vi "Marvin.vi"() -> ()   [LabVIEW 2017]
uses:
  PCAN_Driver/ControlCAN.llb/CAN Channel.ctl
  PCAN_Driver/ControlCAN.llb/DevType.ctl
  PCAN_Driver/ControlCAN.llb/VCI_INIT_CONFIG.ctl
  PCAN_Driver/ControlCAN.llb/InitFlag.ctl
  PCAN_Driver/ControlCAN.llb/Fliter.ctl
  PCAN_Driver/ControlCAN.llb/Mode.ctl
  <vilib>/Utility/miscctls.llb/LVMinMaxIncTypeDef.ctl
  PCAN_Driver/ControlCAN.llb/VCI_CAN_OBJ.ctl
  PCAN_Driver/ControlCAN.lvlib
panel:
  in  "Numeric":i32=100
  in  "Help Button":bool
  in  "Clear Monitor":bool
  out "Array":u64[][](array[numeric]) format="%016x"
  out "Waveform Chart":dbl[](graph)
  out "Ambient Over temp":bool
  out "Ambient Sensor temp":bool
  out "Ambient Temperature":dbl
  in  "Motor Over Temp":bool
  in  "Speed control":bool
  out "Unit Adress":string
  in  "Serial Send":bool
  in  "Index":u16(ring) items=["1"=1, "2"=2, "3"=3]
  out "read buffer":string
  in  "SetGet":enum16{"Get", "Set"}(ring)
  in  "Function":T1(ring)
  in  "Value":dbl
  in  "Value 1/2":enum16{"1", "2"}(ring)
  out "Msg Count":u32
  in  "Param to Set":u16(ring) items=["EBAY 5F"=95, "AHU 3F"=63, "AHU 2F"=47]
  out "UUT":u8
  out "Horizontal Progress Bar":i32(slide) min=0 max=48 scale=0.0..50.0
  in  "Set Param.":bool
  in  "Serial Monitor":bool caption="Graph Button"
  in  "Serial Com":bool
  in  "VISA resource name":refnum<visa-resource-name>="COM6"
  out "Serial Status":bool
  in  "Graph Button":bool
  in  "Refresh Button":bool
  out "Data Send":u64 format="%016x"
  in  "Motor Speed RPM":u16
  out "Under voltage/Over voltage":bool
  out "Speed error":bool
  out "Derated drive temp":bool
  out "Motor Over temperature":bool
  out "Commutation err":bool
  out "Motor Sensor temp Fauilre":bool
  out "Drive Over temperature":bool
  out "Drive Sensor temp Failure":bool
  out "Motor Phase Current RMS":dbl
  out "ECS State":u16
  out "Motor Speed RPM":dbl
  out "Motor Stator Temp.":dbl
  out "Power transistor Heat sink Temp.":dbl
  out "DC Current":dbl
  out "DC Voltage":dbl
  in  "Can Send":bool
  in  "Stop":bool
  out "Config_CANAT":T8 {"DevType" items=["USB-CAN"=3, "USB-CAN2"=4]; "CanIndex" items=["通道1", "通道2"]; "VCI_INIT_CONFIG"."Fliter" items=["接收所有类型"=3, "只接收标准帧"=4, "只接收扩展帧"=7]; "VCI_INIT_CONFIG"."Mode" items=["正常工作", "自测模式（环回）", "仅侦听模式"]; "VCI_INIT_CONFIG"."InitFlag" items=["使用Flash参数", "使用界面设置参数"]}
  in  "Channel 2":T3 caption="Channel" items=["Channel 1", "Channel 2"]
  out "CAN Status":bool
  # "ver 1.5"
  # "Marvin"
  # "REDLER TECHNOLOGIES LTD"
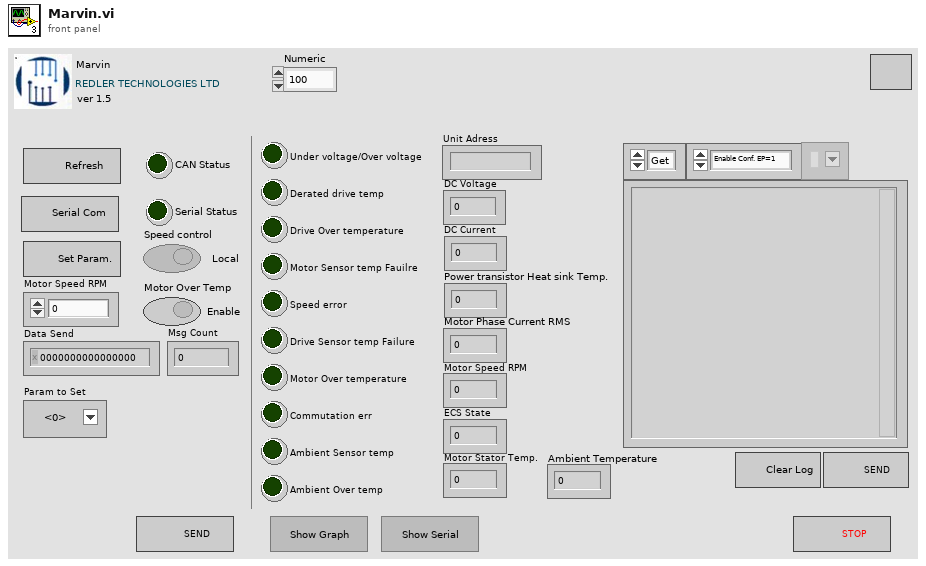
[diagram p1: front panel]
types:
  T1 = enum16{"Enable Conf. EP=1", "Serial Number", "Temperature", "Unit Adress", "Calibration", "Velocity", "Version"}
  T2 = typedef "ControlCAN.lvlib/DevType.ctl" = u32
  T3 = typedef "ControlCAN.lvlib/CAN Channel.ctl" = u32
  T4 = typedef "ControlCAN.lvlib/VCI_INIT_CONFIG.ctl" = cluster{"AccCode":u32, "AccMask":u32, "InitFlag":T5, "Fliter":T6, "Timing0":u8, "Timing1":u8, "Mode":T7}
  T5 = typedef "ControlCAN.lvlib/InitFlag.ctl" = u32
  T6 = typedef "ControlCAN.lvlib/Fliter.ctl" = u8
  T7 = typedef "ControlCAN.lvlib/Mode.ctl" = u8
  T8 = cluster{"DevType":T2, "DevIndex":u32, "CanIndex":T3, "VCI_INIT_CONFIG":T4}
  T9 = cluster{"ID":u32, "MSGTYPE":u8, "LEN":u8, "aDATA":u8[]}[]
  T10 = cluster{"ID":u32, "MSGTYPE":u8, "LEN":u8, "aDATA":u8[]}
  T11 = enum8{"Enabled", "Disabled", "Disabled and Grayed Out"}
  T12 = typedef "LVMinMaxIncTypeDef.ctl" = cluster{"Minimum":dbl, "Maximum":dbl, "Increment":dbl}
  T13 = enum32{"Invalid", "Standard", "Closed", "Hidden", "Minimized", "Maximized"}
  T14 = typedef "ControlCAN.lvlib/VCI_CAN_OBJ.ctl" = cluster{"ID":u32, "TimeStamp":u32, "TimeFlag":u8, "SendType":u8, "RemoteFlag":u8, "ExternFlag":u8, "DataLen":u8, "Data":u8[], "Reserved":u8[]}
  T15 = cluster{"Type":enum16{"接收", "发送"}, "Channel":T3, "Time":timestamp, "VCI_CAN_OBJ":T14}[]
  T16 = cluster{"Type":enum16{"接收", "发送"}, "Channel":T3, "Time":timestamp, "VCI_CAN_OBJ":T14}
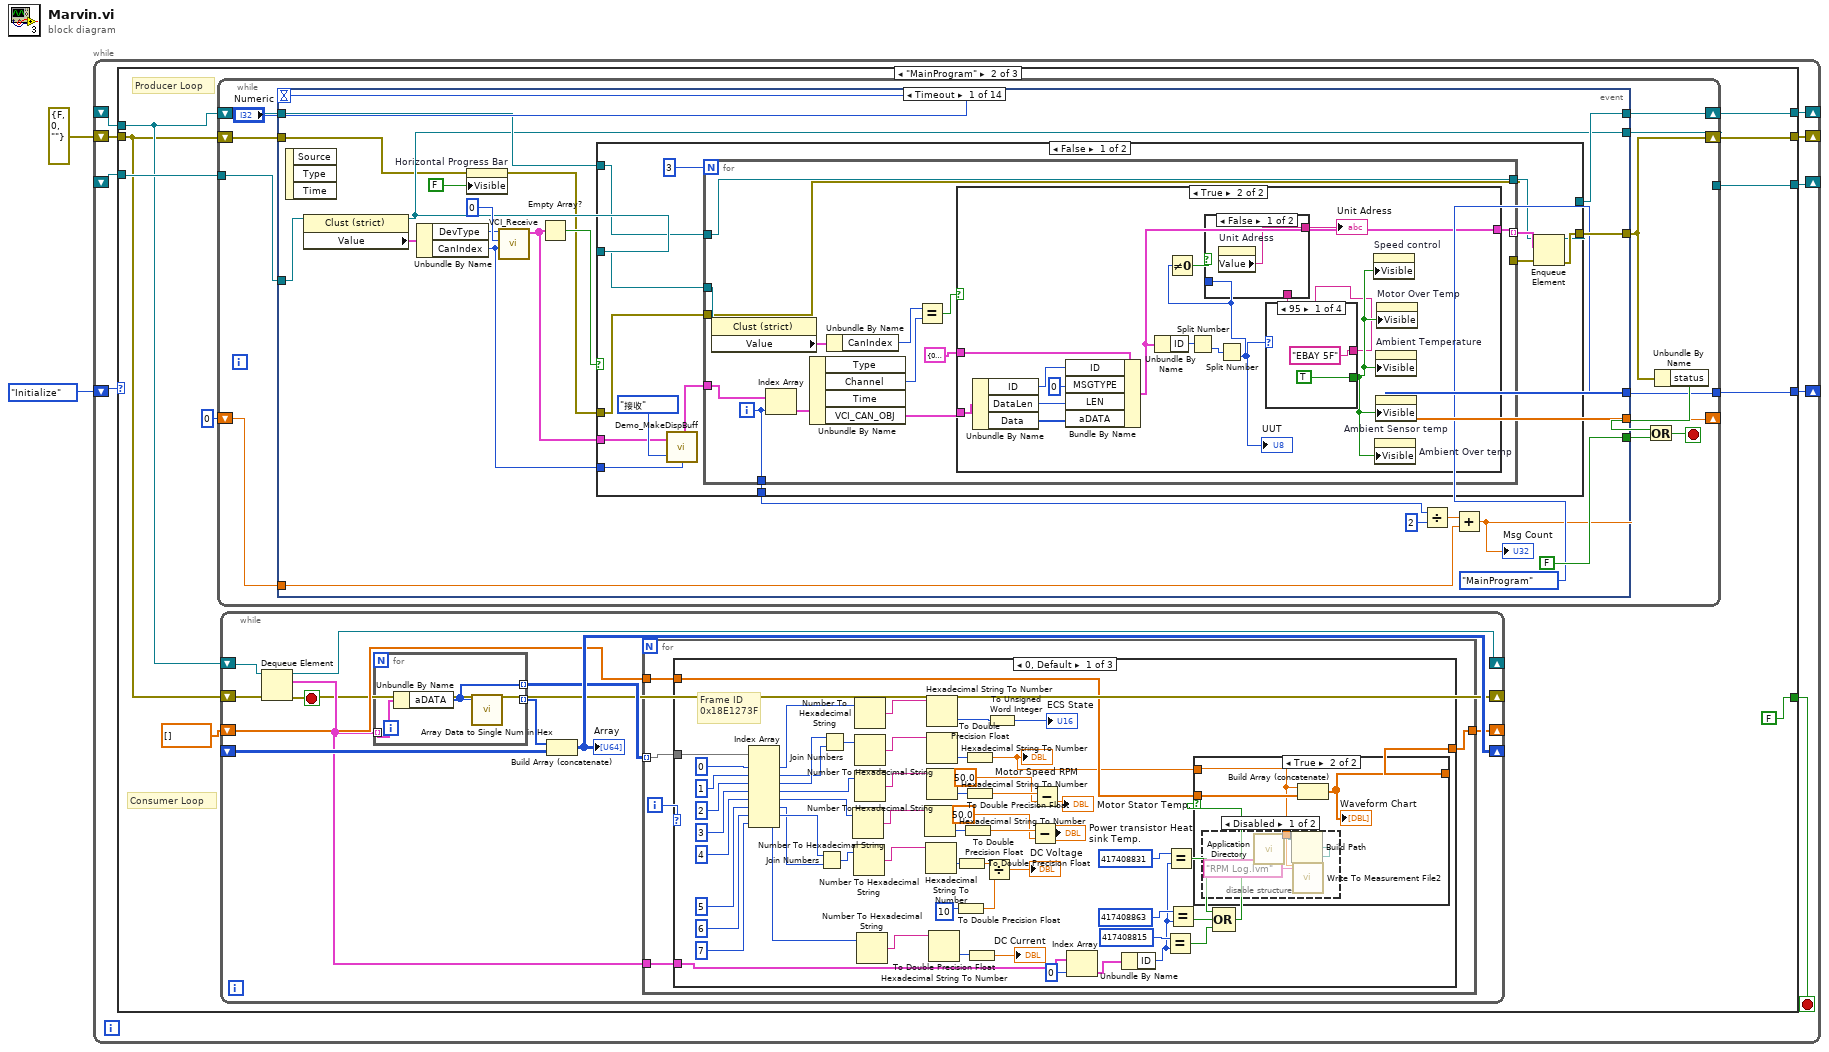
[diagram p0: block diagram]
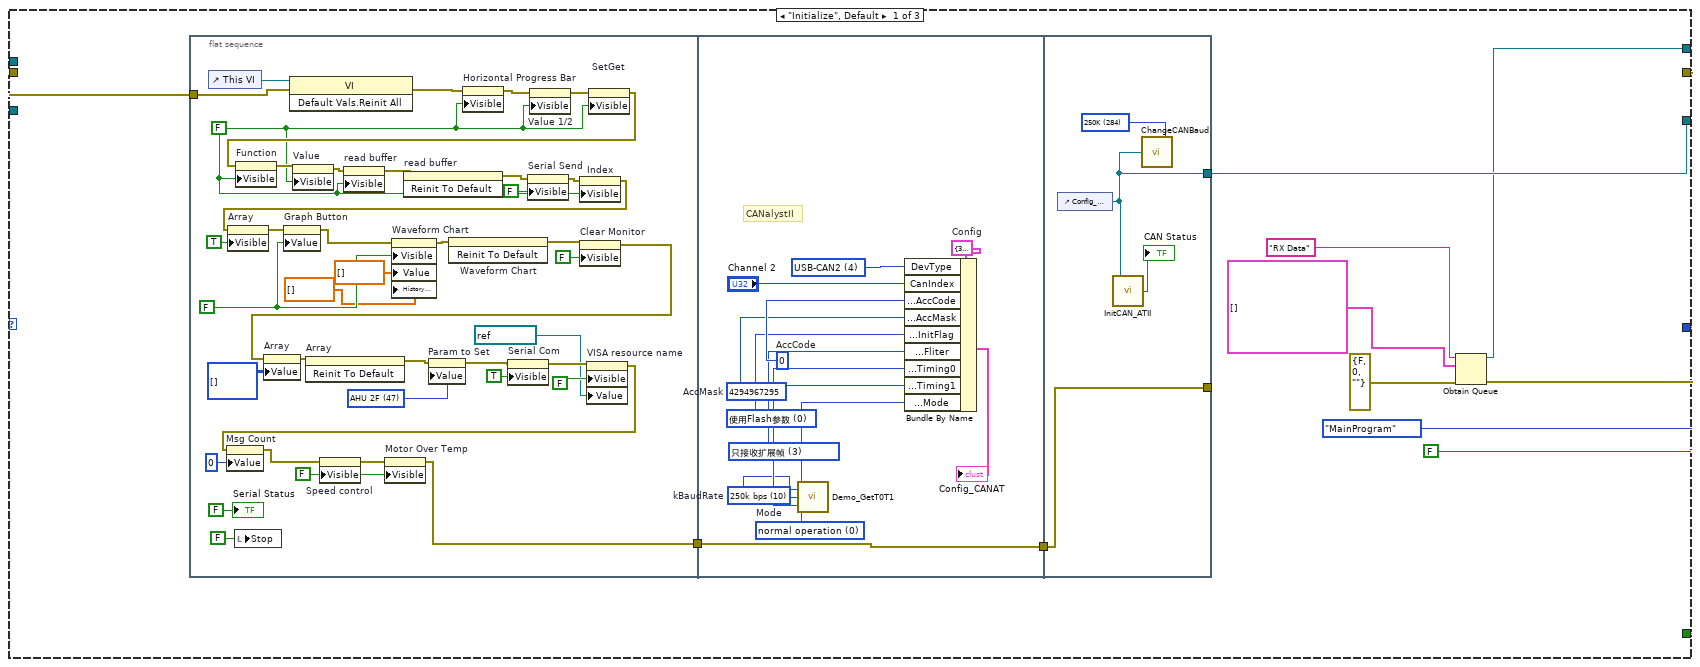
[diagram p2: hidden frame]
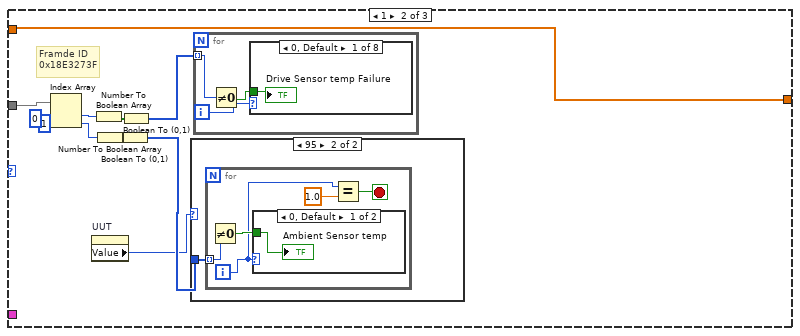
[diagram p5: hidden frame]
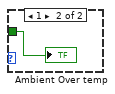
[diagram p7: hidden frame]
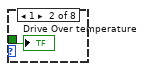
[diagram p8: hidden frame]
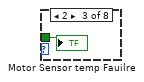
[diagram p9: hidden frame]
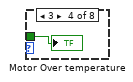
[diagram p10: hidden frame]
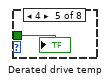
[diagram p11: hidden frame]
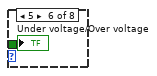
[diagram p12: hidden frame]
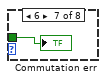
[diagram p13: hidden frame]
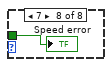
[diagram p14: hidden frame]
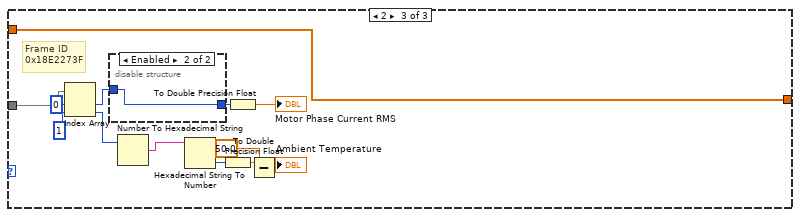
[diagram p15: hidden frame]
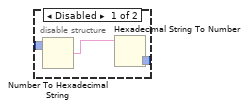
[diagram p16: hidden frame]
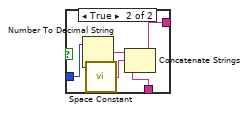
[diagram p18: hidden frame]
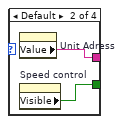
[diagram p19: hidden frame]
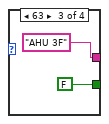
[diagram p20: hidden frame]
diagram:
  n1 = while {
    shift-right: [w6] -> _
    shift-left: enum16{"Stop", "MainProgram", "Initialize"}."Initialize" -> [w11]
    shift-right: [w10] -> _
    shift-left: _ -> [w9]
    shift-right: [w8] -> _
    shift-left: _ -> [w5]
    shift-right: [w7] -> _
    shift-left: errorcluster {"status"=FALSE, "code"=0, "source"=""} ("error out") -> [w4]
    stop <- w3 stop-if-true
    n2 = case shown="\"MainProgram\"" w11 {
      tunnel: [w22 w87 w917] -> w10
      tunnel: w9 -> [_ w90 w917]
      tunnel: [w18 w89 w918] -> w8
      tunnel: [w17 w88 w919] -> w7
      tunnel: [enum16{"Stop", "MainProgram", "Initialize"}."MainProgram" w86 enum16{"Stop", "MainProgram", "Initialize"}."Stop"] -> w6
      tunnel: w5 -> [_ w85 w918]
      tunnel: w4 -> [w15 w84 w920]
      tunnel: [FALSE ("Stop") FALSE ("Stop") w916] -> w3
      frame "Initialize", Default {
        n3 = flat-sequence {
          tunnel: w15 -> [w36]
          tunnel: [w32] -> w13
          tunnel: [w64] -> w14
          tunnel: w13 -> [w64]
          tunnel: [w78] -> w22
          tunnel: w14 -> [w77]
          tunnel: [w77] -> _
          frame #0 {
            w31 = FALSE ("Visible")
            w49 = u16 47 items=["EBAY 5F"=95, "AHU 3F"=63, "AHU 2F"=47] ("Param to Set")
            w26 = FALSE ("Visible")
            w55 = FALSE ("Graph Button")
            n4 = control-ref of="This VI"() -> (w63:refnum<vi>)
            n5 = local write "Stop"(FALSE ("Stop")) -> ()
            n6 = invoke class="VI" method="Default Vals.Reinit All"(reference=w63, error in=w36) -> (error out=w35:errorcluster)  [unwired: 1 in, 2 out]
            n7 = property on="Horizontal Progress Bar" class="Slide (strict)"(error in=w35, "Visible"=w26) -> (error out=w47:errorcluster)  [unwired: 1 in, 1 out]
            n8 = property on="Value 1/2" class="Enum (strict)"(error in=w47, "Visible"=w26) -> (error out=w46:errorcluster)  [unwired: 1 in, 1 out]
            n9 = property on="SetGet" class="Enum (strict)"(error in=w46, "Visible"=w26) -> (error out=w45:errorcluster)  [unwired: 1 in, 1 out]
            n10 = property on="Function" class="Enum (strict)"(error in=w45, "Visible"=w26) -> (error out=w44:errorcluster)  [unwired: 1 in, 1 out]
            n11 = property on="Value" class="DigNum (strict)"(error in=w44, "Visible"=w26) -> (error out=w43:errorcluster)  [unwired: 1 in, 1 out]
            n12 = property on="read buffer" class="Str"(error in=w43, "Visible"=w26) -> (error out=w28:errorcluster)  [unwired: 1 in, 1 out]
            n13 = invoke on="read buffer" class="Str" method="Reinit To Default"(error in=w28) -> (error out=w27:errorcluster)  [unwired: 2 in, 2 out]
            n14 = property on="Serial Send" class="Bool"(error in=w27, "Visible"=FALSE) -> (error out=w42:errorcluster)  [unwired: 1 in, 1 out]
            n15 = property on="Index" class="Ring (strict)"(error in=w42, "Visible"=w26) -> (error out=w41:errorcluster)  [unwired: 1 in, 1 out]
            n16 = property on="Array" class="Arr (strict)"(error in=w41, "Visible"=TRUE) -> (error out=w40:errorcluster)  [unwired: 1 in, 1 out]
            n17 = property on="Graph Button" class="Bool (strict)"(error in=w40, "Value"=w55) -> (error out=w39:errorcluster)  [unwired: 1 in, 1 out]
            n18 = property on="Waveform Chart" class="WFChart (strict)"(error in=w39, "Visible"=w55, "Value"=dbl[] [] ("Waveform Chart"), "History Data"=dbl[] []) -> (error out=w58:errorcluster)  [unwired: 1 in, 1 out]
            n19 = invoke on="Waveform Chart" class="WFChart (strict)" method="Reinit To Default"(error in=w58) -> (error out=w25:errorcluster)  [unwired: 2 in, 2 out]
            n20 = property on="Clear Monitor" class="Bool"(error in=w25, "Visible"=FALSE) -> (error out=w24:errorcluster)  [unwired: 1 in, 1 out]
            n21 = property on="Array" class="Arr (strict)"(error in=w24, "Value"=u64[][] [] ("Array")) -> (error out=w30:errorcluster)  [unwired: 1 in, 1 out]
            n22 = invoke on="Array" class="Arr (strict)" method="Reinit To Default"(error in=w30) -> (error out=w29:errorcluster)  [unwired: 2 in, 2 out]
            n23 = property on="Param to Set" class="Ring (strict)"(error in=w29, "Value"=w49) -> (error out=w38:errorcluster)  [unwired: 1 in, 1 out]
            n24 = property on="Serial Com" class="Bool"(error in=w38, "Visible"=TRUE) -> (error out=w60:errorcluster)  [unwired: 1 in, 1 out]
            n25 = property on="VISA resource name" class="VISAName"(error in=w60, "Visible"=FALSE, "Value"=refnum<visa-resource-name> "COM1" ("VISA resource name")) -> (error out=w37:errorcluster)  [unwired: 1 in, 1 out]
            n26 = property on="Msg Count" class="DigNum (strict)"(error in=w37, "Value"=u32 0 ("Msg Count")) -> (error out=w34:errorcluster)  [unwired: 1 in, 1 out]
            n27 = property on="Speed control" class="Bool (strict)"(error in=w34, "Visible"=w31) -> (error out=w33:errorcluster)  [unwired: 1 in, 1 out]
            n28 = property on="Motor Over Temp" class="Bool (strict)"(error in=w33, "Visible"=w31) -> (error out=w32:errorcluster)  [unwired: 1 in, 1 out]
            "Serial Status" <- FALSE ("Serial Status")
          }
          frame #1 {
            w68 = u32 4294967295  # AccMask
            w67 = T5 0 items=["使用Flash参数", "使用界面设置参数"] ("InitFlag")
            w65 = T7 0 items=["normal operation", "Listen-only mode", "test mode"]  # Mode
            w66 = T6 3 items=["接收所有类型"=1, "只接收标准帧"=2, "只接收扩展帧"=3] ("Fliter")
            w72 = u8 10 items=["5k bps"=1, "10k bps"=2, "20k bps"=3, "40k bps"=4, "50k bps"=5, "80k bps"=6, "100k bps"=7, "125k bps"=8, "200k bps"=9, "250k bps"=10, "400k bps"=11, "500k bps"=12, "666k bps"=13, "800k bps"=14, "1000k bps"=15, "33.33k bps"=16, "66.66k bps"=17, "83.33k bps"=18]  # kBaudRate
            w69 = u32 0  # AccCode
            w70 = T2 4 items=["USB-CAN"=3, "USB-CAN2"=4] ("DevType")
            w71 = T8 {"DevType"=3, "DevIndex"=0, "CanIndex"=0, "VCI_INIT_CONFIG"={"AccCode"=0, "AccMask"=0, "InitFlag"=1, "Fliter"=7, "Timing0"=0, "Timing1"=0, "Mode"=0}}  # Config
            # "CANalystII"
            n29 = call "Demo_GetT0T1.vi"("kBaudRate"=w72) -> ("Timing0"=w74:u8, "Timing1"=w75:u8)
            n30 = Bundle By Name(cluster=w71, "DevType"=w70, "CanIndex"="Channel 2", "VCI_INIT_CONFIG.AccCode"=w69, "VCI_INIT_CONFIG.AccMask"=w68, "VCI_INIT_CONFIG.InitFlag"=w67, "VCI_INIT_CONFIG.Fliter"=w66, "VCI_INIT_CONFIG.Timing0"=w74, "VCI_INIT_CONFIG.Timing1"=w75, "VCI_INIT_CONFIG.Mode"=w65) -> (→"Config_CANAT":T8)
          }
          frame #2 {
            w79 = u16 284 items=["1M"=20, "500K"=28, "250K"=284, "125K"=796, "100K"=17199, "50K"=18223, "20K"=21295, "10K"=26415, "5K"=32639] ("baud in")
            n31 = control-ref of="Config_CANAT"() -> (w78:refnum<vi>)
            n32 = call "InitCAN_ATII.vi"("Config"=w78) -> ("Sts"=→"CAN Status":bool)
            n33 = call "ChangeCANBaud.vi"("baud in"=w79, "reference"=w78) -> ()
          }
        }
        n34 = Obtain Queue(name (unnamed)="RX Data", element data type=T9 [], error in (no error)=errorcluster {"status"=FALSE, "code"=0, "source"=""}) -> (queue out=w18:refnum<queue>, error out=w17:errorcluster)  [unwired: 2 in, 1 out]
      }
      frame "MainProgram" {
        # "Consumer Loop"
        # "Producer Loop"
        n35 = while {
          shift-right: [w228] -> w88
          shift-left: w84 -> [w230]
          shift-right: [w229] -> w89
          shift-left: w85 -> [w231]
          tunnel: w90 -> [w232]
          tunnel: [w225] -> w87
          tunnel: [w224] -> w86
          shift-right: [w222] -> _
          shift-left: 0 -> [w223]
          stop <- w233 stop-if-true
          n36 = event shown="[0] Timeout" {
            selector: _ -> [_ _ _ _ _ _ _ _ _ _ _ _ _ _]
            dyn-events: _ -> [_ _ _ _ _ _ _ _ _ _ _ _ _ _]
            timeout: "Numeric" -> [_ _ _ _ _ _ _ _ _ _ _ _ _ _]
            tunnel: w232 -> [w252 w322 w332 w392 w582 w615 w662 w759 w779 w855 w875 w892 w907 w913]
            tunnel: w231 -> [w249 w323 w335 w393 w583 w616 w661 w760 w800 w856 w874 w893 w904 w910]
            tunnel: w230 -> [w241 w321 w330 w387 w585 w618 w654 w752 w799 w848 w870 w885 w903 w911]
            tunnel: [w247 w323 w335 w393 w583 w616 w661 w760 w800 w856 w874 w893 w902 w910] -> w229
            tunnel: [w246 w315 w331 w384 w581 w617 w650 w749 w799 w836 w867 w883 w900 w909] -> w228
            tunnel: [FALSE ("Stop") FALSE ("Stop") FALSE ("Stop") FALSE ("Stop") FALSE ("Stop") FALSE ("Stop") FALSE ("Stop") FALSE ("Stop") FALSE ("Stop") FALSE ("Stop") FALSE ("Stop") FALSE ("Stop") TRUE ("Stop") TRUE ("Stop")] -> w226
            tunnel: [w245 w322 w332 w392 w582 w615 w662 w759 w779 w855 w875 w892 w907 w913] -> w225
            tunnel: [enum16{"Stop", "MainProgram", "Initialize"}."MainProgram" enum16{"Stop", "MainProgram", "Initialize"}."MainProgram" enum16{"Stop", "MainProgram", "Initialize"}."MainProgram" enum16{"Stop", "MainProgram", "Initialize"}."MainProgram" enum16{"Stop", "MainProgram", "Initialize"}."MainProgram" enum16{"Stop", "MainProgram", "Initialize"}."MainProgram" enum16{"Stop", "MainProgram", "Initialize"}."MainProgram" enum16{"Stop", "MainProgram", "Initialize"}."MainProgram" enum16{"Stop", "MainProgram", "Initialize"}."MainProgram" enum16{"Stop", "MainProgram", "Initialize"}."MainProgram" enum16{"Stop", "MainProgram", "Initialize"}."MainProgram" enum16{"Stop", "MainProgram", "Initialize"}."MainProgram" enum16{"Stop", "MainProgram", "Initialize"}."Stop" enum16{"Stop", "MainProgram", "Initialize"}."Initialize"] -> w224
            tunnel: w223 -> [w240 w326 w328 w380 w579 w614 w652 w763 w765 w846 w866 w881 w899 w908]
            tunnel: [w239 w326 w328 w380 w579 w614 w652 w763 w765 w846 w866 w881 w899 w908] -> w222
            event Timeout {
              n37 = event-data() -> ()  [unwired: 1 in, 3 out]
              n38 = property class="Clust (strict)"(reference=w252) -> (reference out=w245:refnum<vi>, "Value"=w253:T8)  [unwired: 1 in, 1 out]
              n39 = Unbundle By Name(w253) -> ("DevType"=w254:T2, "CanIndex"=w250:T3)
              n40 = property on="Horizontal Progress Bar" class="Slide (strict)"(error in=w241, "Visible"=FALSE) -> (error out=w235:errorcluster)  [unwired: 1 in, 1 out]
              n41 = call "VCI_Receive.vi"("CANIndex"=w250, "DevIndex"=u32 0, "DevType"=w254) -> ("Recieve"=w248:T14[])  [unwired: 3 in, 5 out]
              n42 = Empty Array?(array=w248) -> (empty?=w251:bool)
              n43 = case shown="False" w251 {
                tunnel: w250 -> [w267 _]
                tunnel: w245 -> [w265 _]
                tunnel: w249 -> [w264 w314]
                tunnel: w235 -> [w263 w313]
                tunnel: w248 -> [w268 _]
                tunnel: [w258 w313] -> w246
                tunnel: [w257 w314] -> w247
                tunnel: [w256 0] -> w236
                frame False {
                  n44 = call "Demo_MakeDispBuff.vi"("Channel"=w267, "Type"=enum16{"接收", "发送"}."接收", "OBJs"=w268) -> ("Buffer"=w266:T15)
                  n45 = for {
                    N: 3 -> [_]
                    tunnel: w266 -> [w282]
                    tunnel: w265 -> [w281]
                    tunnel: w264 -> [w272]
                    tunnel: w263 -> [w271]
                    tunnel: [w274] -> w261 mode=indexing
                    tunnel: [w272] -> w260
                    tunnel: [w271] -> w259
                    tunnel: [w270] -> w256
                    i -> [w270]
                    n46 = property class="Clust (strict)"(reference=w281) -> ("Value"=w279:T8)  [unwired: 1 in, 2 out]
                    n47 = Index Array(array=w282, index=w270) -> (element=w275:T16)
                    n48 = Unbundle By Name(w275) -> ("Channel"=w277:T3, "VCI_CAN_OBJ"=w280:T14)  [unwired: 2 out]
                    n49 = Unbundle By Name(w279) -> ("CanIndex"=w278:T3)
                    n50 = Equal?(x=w278, y=w277) -> (x = y?=w276:bool)
                    n51 = case shown="True" w276 {
                      tunnel: w280 -> [_ w297]
                      tunnel: [w283 w293] -> w274
                      tunnel: T10 {"ID"=0, "MSGTYPE"=0, "LEN"=0, "aDATA"=[]} ("Msg") -> [w283 w292]
                      frame False {
                      }
                      frame True {
                        n52 = Unbundle By Name(w297) -> ("ID"=w291:u32, "DataLen"=w296:u8, "Data"=w294:u8[])
                        n53 = Bundle By Name(cluster=w292, "ID"=w291, "MSGTYPE"=u8 0, "LEN"=w296, "aDATA"=w294) -> (w293:T10)
                        n54 = Unbundle By Name(w293) -> ("ID"=w289:u32)
                        n55 = Split Number(x=w289) -> (lo(x)=w290:u16)  [unwired: 1 out]
                        n56 = Split Number(x=w290) -> (lo(x)=w286:u8)  [unwired: 1 out]
                        "UUT" <- w286
                        n57 = Not Equal To 0?(x=w286) -> (x != 0?=w287:bool)
                        n58 = case shown="95" w286 {
                          tunnel: ["EBAY 5F" w306 "AHU 3F" "AHU 2F"] -> w285
                          tunnel: [TRUE w307 FALSE FALSE] -> w288
                          frame 95 {
                          }
                          frame Default {
                            n59 = property on="Unit Adress" class="Str"() -> ("Value"=w306:string)  [unwired: 2 in, 2 out]
                            n60 = property on="Speed control" class="Bool (strict)"() -> ("Visible"=w307:bool)  [unwired: 2 in, 2 out]
                          }
                          frame 63 {
                          }
                          frame 47 {
                          }
                        }
                        n61 = case shown="False" w287 {
                          tunnel: w286 -> [_ w303]
                          tunnel: w285 -> [_ w300]
                          tunnel: [w298 w299] -> w284
                          frame False {
                            n62 = property on="Unit Adress" class="Str"() -> ("Value"=w298:string)  [unwired: 2 in, 2 out]
                          }
                          frame True {
                            n63 = Number To Decimal String(number=w303) -> (decimal integer string=w302:string)  [unwired: 1 in]
                            n64 = call <vilib>:"Space Constant.vi"() -> ("String"=w301:string)
                            n65 = Concatenate Strings(w302, w301, w300) -> (w299:string)
                          }
                        }
                        "Unit Adress" <- w284
                        n66 = property on="Speed control" class="Bool (strict)"("Visible"=w288) -> ()  [unwired: 2 in, 2 out]
                        n67 = property on="Ambient Over temp" class="Bool (strict)"("Visible"=w288) -> ()  [unwired: 2 in, 2 out]
                        n68 = property on="Ambient Temperature" class="DigNum (strict)"("Visible"=w288) -> ()  [unwired: 2 in, 2 out]
                        n69 = property on="Ambient Sensor temp" class="Bool (strict)"("Visible"=w288) -> ()  [unwired: 2 in, 2 out]
                        n70 = property on="Motor Over Temp" class="Bool (strict)"("Visible"=w288) -> ()  [unwired: 2 in, 2 out]
                      }
                    }
                  }
                  n71 = Enqueue Element(queue=w260, element=w261, error in (no error)=w259) -> (queue out=w257:refnum<queue>, error out=w258:errorcluster)  [unwired: 2 out]
                }
                frame True {
                }
              }
              n72 = Divide(x=w236, y=u32 2) -> (x/y=w237:dbl)
              n73 = Add(x=w237, y=w240) -> (x+y=w239:dbl)
              "Msg Count" <- w239
            }
            event "Clear Monitor": Value Change {
              n74 = event-data() -> ()  [unwired: 1 in, 6 out]
              n75 = property on="VISA resource name" class="VISAName"(error in=w321) -> (error out=w320:errorcluster, "Value"=w318:refnum<visa-resource-name>)  [unwired: 1 in, 1 out]
              n76 = call "Serial.vi"("error in (no error)"=w320, "Clear Log"=TRUE, "VISA resource name"=w318) -> ("error out"=w316:errorcluster, "read buffer"=w317:string)  [unwired: 6 in, 1 out]
              n77 = property on="read buffer" class="Str"(error in=w316, "Value"=w317) -> (error out=w315:errorcluster)  [unwired: 1 in, 1 out]
            }
            event "Serial Monitor": Value Change {
              n78 = event-data() -> ()  [unwired: 1 in, 6 out]
              n79 = property on="Serial Status" class="Bool (strict)"(error in=w330) -> (error out=w329:errorcluster, "Value"=w327:bool)  [unwired: 1 in, 1 out]
              n80 = case shown="True" w327 {
                tunnel: w329 -> [w339 w352]
                tunnel: [w337 w357] -> w331
                frame False {
                  n81 = call "Display Message to User3"("error in (no error)"=w339) -> ("error out"=w338:errorcluster)  [unwired: 9 in, 1 out]
                  n82 = property on="Serial Monitor" class="Bool (strict)"(error in=w338, "Value"=FALSE ("Serial Monitor")) -> (error out=w337:errorcluster)  [unwired: 1 in, 1 out]
                }
                frame True {
                  w344 = FALSE ("Visible")
                  w354 = FALSE ("Visible")
                  w355 = u16 1 items=["1"=1, "2"=2, "3"=3] ("Index")
                  n83 = property on="Index" class="Ring (strict)"(error in=w352, "Value"=w355) -> (error out=w351:errorcluster)  [unwired: 1 in, 1 out]
                  n84 = property on="Value 1/2" class="Enum (strict)"(error in=w351, "Visible"=w354) -> (error out=w350:errorcluster)  [unwired: 1 in, 1 out]
                  n85 = property on="Value" class="DigNum (strict)"(error in=w350, "Visible"=w354) -> (error out=w349:errorcluster)  [unwired: 1 in, 1 out]
                  n86 = property on="SetGet" class="Enum (strict)"(error in=w349, "Value"=enum16{"Get", "Set"}."Get" ("SetGet")) -> (error out=w348:errorcluster)  [unwired: 1 in, 1 out]
                  n87 = property on="Serial Send" class="Bool"(error in=w348, "Visible"=w344) -> (error out=w343:errorcluster)  [unwired: 1 in, 1 out]
                  n88 = property on="Clear Monitor" class="Bool"(error in=w343, "Visible"=w344) -> (error out=w342:errorcluster)  [unwired: 1 in, 1 out]
                  n89 = property on="Function" class="Enum (strict)"(error in=w342, "Value"=T1."Serial Number" ("Function")) -> (error out=w347:errorcluster)  [unwired: 1 in, 1 out]
                  n90 = property on="Index" class="Ring (strict)"(error in=w347, "DisabledEnum"=T11."Disabled and Grayed Out" ("Disabled")) -> (error out=w345:errorcluster)  [unwired: 1 in, 1 out]
                  n91 = case shown="True" "Serial Monitor" {
                    selector: "Serial Monitor" -> [w361 w376]
                    tunnel: w345 -> [w360 w379]
                    tunnel: [w363 w373] -> w357
                    tunnel: [FALSE TRUE] -> w341
                    frame False {
                      n92 = property on="Graph Button" class="Bool (strict)"(error in=w360) -> (error out=w359:errorcluster, "Value"=w358:bool)  [unwired: 1 in, 1 out]
                      n93 = case shown="True" w358 {
                        tunnel: [w368 w371] -> w364
                        tunnel: w359 -> [w367 w370]
                        tunnel: w361 -> [w365 _]
                        frame False {
                          n94 = Not(x=w365) -> (.not. x?=w366:bool)
                          n95 = property on="Array" class="Arr (strict)"(error in=w367, "Visible"=w366) -> (error out=w368:errorcluster)  [unwired: 1 in, 1 out]
                        }
                        frame True {
                          n96 = property on="Array" class="Arr (strict)"(error in=w370, "Visible"=FALSE) -> (error out=w371:errorcluster)  [unwired: 1 in, 1 out]
                        }
                      }
                      n97 = property on="Serial Monitor" class="Bool (strict)"(error in=w364, "Value"=w361) -> (error out=w363:errorcluster)  [unwired: 1 in, 1 out]
                    }
                    frame True {
                      n98 = Not(x=w376) -> (.not. x?=w372:bool)
                      n99 = property on="Array" class="Arr (strict)"(error in=w379, "Visible"=w372) -> (error out=w378:errorcluster)  [unwired: 1 in, 1 out]
                      n100 = property on="Serial Monitor" class="Bool (strict)"(error in=w378, "Value"=w376) -> (error out=w375:errorcluster)  [unwired: 1 in, 1 out]
                      n101 = property on="Graph Button" class="Bool (strict)"(error in=w375, "Value"=w372) -> (error out=w374:errorcluster)  [unwired: 1 in, 1 out]
                      n102 = property on="Waveform Chart" class="WFChart (strict)"(error in=w374, "Visible"=w372) -> (error out=w373:errorcluster)  [unwired: 1 in, 1 out]
                    }
                  }
                  n103 = property on="SetGet" class="Enum (strict)"("Visible"=w341) -> ()  [unwired: 2 in, 2 out]
                  n104 = property on="Index" class="Ring (strict)"("Visible"=w341) -> ()  [unwired: 2 in, 2 out]
                  n105 = property on="Function" class="Enum (strict)"("Visible"=w341) -> ()  [unwired: 2 in, 2 out]
                  n106 = property on="Clear Monitor" class="Bool"("Visible"=w341) -> ()  [unwired: 2 in, 2 out]
                  n107 = property on="Serial Send" class="Bool"("Visible"=w341) -> ()  [unwired: 2 in, 2 out]
                  n108 = property on="read buffer" class="Str"("Visible"=w341) -> ()  [unwired: 2 in, 2 out]
                }
              }
            }
            event "Serial Send": Value Change {
              n109 = event-data() -> ()  [unwired: 1 in, 6 out]
              n110 = property on="read buffer" class="Str"(error in=w387) -> (error out=w386:errorcluster, "Text.Scroll Position"=w383:u32)  [unwired: 1 in, 1 out]
              n111 = property on="VISA resource name" class="VISAName"() -> ("Value"=w394:refnum<visa-resource-name>)  [unwired: 2 in, 2 out]
              n112 = case shown="\"Get\", Default" "SetGet" {
                tunnel: "Function" -> [w401 w486]
                tunnel: w394 -> [w407 w499]
                tunnel: w386 -> [w404 w485]
                tunnel: "Value" -> [_ w498]
                tunnel: "Value 1/2" -> [_ w496]
                tunnel: "Index" -> [w402 w493]
                tunnel: [w406 w491] -> w385
                tunnel: [w399 w489] -> w391
                frame "Get", Default {
                  w405 = FALSE ("Visible")
                  n113 = property on="Value" class="DigNum (strict)"(error in=w404, "Visible"=w405) -> (error out=w403:errorcluster)  [unwired: 1 in, 1 out]
                  n114 = property on="Value 1/2" class="Enum (strict)"(error in=w403, "Visible"=w405) -> (error out=w400:errorcluster)  [unwired: 1 in, 1 out]
                  n115 = case shown="\"Temperature\"" w401 {
                    tunnel: w407 -> [w412 w430 w446 w455 w462 w473]
                    tunnel: w400 -> [w410 w421 w436 w450 w460 w471]
                    tunnel: [w415 w431 w447 w456 w466 w474] -> w406
                    tunnel: [w414 w432 w445 w457 w467 w469] -> w399
                    tunnel: w402 -> [_ w425 w438 _ _ _]
                    frame "Serial Number", Default {
                      n116 = Concatenate Strings("SN" ("string"), "\r\n" ("write buffer")) -> (w413:string)
                      n117 = property on="Index" class="Ring (strict)"(error in=w410, "DisabledEnum"=T11."Disabled and Grayed Out" ("Disabled")) -> (error out=w409:errorcluster)  [unwired: 1 in, 1 out]
                      n118 = call "Serial.vi"("error in (no error)"=w409, "Clear Log"=FALSE, "write buffer"=w413, "VISA resource name"=w412) -> ("error out"=w415:errorcluster, "read buffer"=w414:string)  [unwired: 5 in, 1 out]
                    }
                    frame "Temperature" {
                      n119 = Number To Decimal String(number=w425) -> (decimal integer string=w424:string)  [unwired: 1 in]
                      n120 = property on="Index" class="Ring (strict)"(error in=w421, "DisabledEnum"=T11."Enabled" ("Disabled"), "Visible"=TRUE) -> (error out=w420:errorcluster)  [unwired: 1 in, 1 out]
                      n121 = Concatenate Strings("TA" ("string"), "[", w424, "]", "\r\n" ("write buffer")) -> (w426:string)
                      n122 = call "Serial.vi"("error in (no error)"=w420, "Clear Log"=FALSE, "write buffer"=w426, "VISA resource name"=w430) -> ("error out"=w431:errorcluster, "read buffer"=w432:string)  [unwired: 5 in, 1 out]
                    }
                    frame "Unit Adress" {
                      n123 = Number To Decimal String(number=w438) -> (decimal integer string=w444:string)  [unwired: 1 in]
                      n124 = property on="Index" class="Ring (strict)"(error in=w436, "DisabledEnum"=T11."Enabled" ("Disabled"), "Visible"=TRUE) -> (error out=w435:errorcluster)  [unwired: 1 in, 1 out]
                      n125 = Concatenate Strings("UA" ("string"), "[", w444, "]", "\r\n" ("write buffer")) -> (w439:string)
                      n126 = call "Serial.vi"("error in (no error)"=w435, "Clear Log"=FALSE, "write buffer"=w439, "VISA resource name"=w446) -> ("error out"=w447:errorcluster, "read buffer"=w445:string)  [unwired: 5 in, 1 out]
                    }
                    frame "Calibration" {
                      n127 = Concatenate Strings("CC" ("string"), "\r\n" ("write buffer")) -> (w453:string)
                      n128 = property on="Index" class="Ring (strict)"(error in=w450, "DisabledEnum"=T11."Disabled and Grayed Out" ("Disabled")) -> (error out=w449:errorcluster)  [unwired: 1 in, 1 out]
                      n129 = call "Serial.vi"("error in (no error)"=w449, "Clear Log"=FALSE, "write buffer"=w453, "VISA resource name"=w455) -> ("error out"=w456:errorcluster, "read buffer"=w457:string)  [unwired: 5 in, 1 out]
                    }
                    frame "Velocity" {
                      n130 = Concatenate Strings("VC" ("string"), "\r\n" ("write buffer")) -> (w463:string)
                      n131 = property on="Index" class="Ring (strict)"(error in=w460, "DisabledEnum"=T11."Disabled and Grayed Out" ("Disabled")) -> (error out=w459:errorcluster)  [unwired: 1 in, 1 out]
                      n132 = call "Serial.vi"("error in (no error)"=w459, "Clear Log"=FALSE, "write buffer"=w463, "VISA resource name"=w462) -> ("error out"=w466:errorcluster, "read buffer"=w467:string)  [unwired: 5 in, 1 out]
                    }
                    frame "Version" {
                      n133 = Concatenate Strings("VR" ("string"), "\r\n" ("write buffer")) -> (w475:string)
                      n134 = property on="Index" class="Ring (strict)"(error in=w471, "DisabledEnum"=T11."Disabled and Grayed Out" ("Disabled")) -> (error out=w470:errorcluster)  [unwired: 1 in, 1 out]
                      n135 = call "Serial.vi"("error in (no error)"=w470, "Clear Log"=FALSE, "write buffer"=w475, "VISA resource name"=w473) -> ("error out"=w474:errorcluster, "read buffer"=w469:string)  [unwired: 5 in, 1 out]
                    }
                  }
                }
                frame "Set" {
                  n136 = To Unsigned Long Integer(number=w498) -> (unsigned 32bit integer=w494:u32)
                  n137 = Number To Decimal String(number=w493) -> (decimal integer string=w492:string)  [unwired: 1 in]
                  n138 = Number To Decimal String(number=w496) -> (decimal integer string=w495:string)  [unwired: 1 in]
                  n139 = case shown="\"Version\"" w486 {
                    tunnel: w485 -> [w506 w510 w514 w518 w522 w526]
                    tunnel: [FALSE TRUE TRUE FALSE FALSE FALSE] -> w483
                    tunnel: [TRUE TRUE TRUE FALSE TRUE FALSE] -> w482
                    tunnel: [FALSE FALSE FALSE TRUE FALSE FALSE] -> w481
                    tunnel: [w506 w510 w514 w518 w522 w526] -> w479
                    frame "Serial Number", Default {
                    }
                    frame "Temperature" {
                    }
                    frame "Unit Adress" {
                    }
                    frame "Calibration" {
                    }
                    frame "Velocity" {
                    }
                    frame "Version" {
                    }
                  }
                  n140 = Number To Decimal String(number=w494) -> (decimal integer string=w497:string)  [unwired: 1 in]
                  n141 = flat-sequence {
                    tunnel: [w529] -> w501
                    tunnel: w478 -> [w529]
                    frame #0 {
                      n142 = Wait (ms)(milliseconds to wait=u32 50) -> ()  [unwired: 1 out]
                    }
                  }
                  n143 = property on="Index" class="Ring (strict)"(error in=w479, "Visible"=w483) -> (error out=w484:errorcluster)  [unwired: 1 in, 1 out]
                  n144 = property on="Value" class="DigNum (strict)"(error in=w484, "Visible"=w482) -> (error out=w480:errorcluster)  [unwired: 1 in, 1 out]
                  n145 = property on="Value 1/2" class="Enum (strict)"(error in=w480, "Visible"=w481) -> (error out=w478:errorcluster)  [unwired: 1 in, 1 out]
                  n146 = case shown="\"Unit Adress\"" w486 {
                    tunnel: [w532 w538 w547 w555 w573 "EP=1\r\n" ("write buffer")] -> w487
                    tunnel: w501 -> [w531 w537 w546 w560 w564 w576]
                    tunnel: [w531 w537 w546 w560 w561 w576] -> w500
                    tunnel: w497 -> [w533 w539 w552 _ _ _]
                    tunnel: w495 -> [_ _ _ w556 _ _]
                    tunnel: w494 -> [_ _ _ _ w565 _]
                    tunnel: w492 -> [_ w540 w550 _ _ _]
                    frame "Serial Number", Default {
                      n147 = Concatenate Strings("SN" ("write buffer"), "=" ("string"), w533, "\r\n" ("write buffer")) -> (w532:string)
                    }
                    frame "Temperature" {
                      n148 = Concatenate Strings("TA" ("string"), "[", w540, "]", "=" ("string"), w539, "\r\n" ("write buffer")) -> (w538:string)
                    }
                    frame "Unit Adress" {
                      n149 = Concatenate Strings("UA" ("string"), "[", w550, "]", "=" ("string"), w552, "\r\n" ("write buffer")) -> (w547:string)
                    }
                    frame "Calibration" {
                      n150 = Concatenate Strings("CC" ("string"), "=" ("string"), w556, "\r\n" ("write buffer")) -> (w555:string)
                    }
                    frame "Velocity" {
                      n151 = In Range and Coerce(upper limit=u16 18001, x=w565, lower limit=u16 0) -> (coerced(x)=w571:u32, In Range?=w569:bool)
                      n152 = Not(x=w569) -> (.not. x?=w570:bool)
                      n153 = Select(t=w571, s=w569, f=u16 0) -> (s? t:f=w563:u32)
                      n154 = call "Display Message to User2"("error in (no error)"=w564, "Enable"=w570) -> ("error out"=w561:errorcluster)  [unwired: 8 in, 1 out]
                      n155 = Number To Decimal String(number=w563) -> (decimal integer string=w562:string)  [unwired: 1 in]
                      n156 = Concatenate Strings("VC" ("write buffer"), "=" ("string"), w562, "\r\n" ("write buffer")) -> (w573:string)
                    }
                    frame "Enable Conf. EP=1" {
                    }
                  }
                  n157 = VISA Write(VISA resource name=w499, write buffer=w487, error in (no error)=w500) -> (error out=w502:errorcluster)  [unwired: 2 out]
                  n158 = flat-sequence {
                    tunnel: w502 -> [w527]
                    tunnel: [w527] -> w491
                    frame #0 {
                      n159 = Wait (ms)(milliseconds to wait=u32 50) -> ()  [unwired: 1 out]
                    }
                  }
                  n160 = feedback #1("") -> (w488:string)
                  n161 = Concatenate Strings(w488, w487) -> (w489:string)
                  n162 = feedback-in #1(w489) -> ()
                }
              }
              "read buffer" <- w391
              n163 = Add(x=u32 5, y=w383) -> (x+y=w382:u32)
              n164 = property on="read buffer" class="Str"(error in=w385, "Text.Scroll Position"=w382) -> (error out=w384:errorcluster)  [unwired: 1 in, 1 out]
            }
            event "Function": Value Change {
              n165 = event-data() -> ("CtlRef"=w587:refnum<vi>)  [unwired: 1 in, 5 out]
              n166 = property class="Enum (strict)"(reference=w587, error in=w585) -> (error out=w584:errorcluster, "Value"=w586:T1)  [unwired: 1 out]
              n167 = case shown="\"Temperature\"" w586 {
                tunnel: w584 -> [w589 w594 w601 w603 w606 w610]
                tunnel: [w588 w596 w600 w605 w608 w609] -> w581
                frame "Serial Number", Default {
                  n168 = property on="Index" class="Ring (strict)"(error in=w589, "DisabledEnum"=T11."Disabled and Grayed Out" ("Disabled")) -> (error out=w588:errorcluster)  [unwired: 1 in, 1 out]
                }
                frame "Temperature" {
                  n169 = property on="UUT" class="DigNum (strict)"() -> ("Value"=w591:u8)  [unwired: 2 in, 2 out]
                  n170 = case shown="95" w591 {
                    tunnel: [i32[] [2] ("Disabled Items []") i32[] [3] ("Disabled Items []")] -> w592
                    frame 47, 63, Default {
                    }
                    frame 95 {
                    }
                  }
                  n171 = property on="Index" class="Ring (strict)"(error in=w594, "DisabledEnum"=T11."Enabled" ("Disabled"), "Visible"=TRUE, "Disabled Items []"=w592) -> (error out=w596:errorcluster)  [unwired: 1 in, 1 out]
                }
                frame "Unit Adress" {
                  n172 = property on="Index" class="Ring (strict)"(error in=w601, "DisabledEnum"=T11."Enabled" ("Disabled"), "Visible"=TRUE) -> (error out=w600:errorcluster)  [unwired: 1 in, 1 out]
                }
                frame "Calibration" {
                  n173 = property on="Index" class="Ring (strict)"(error in=w603, "DisabledEnum"=T11."Disabled and Grayed Out" ("Disabled")) -> (error out=w605:errorcluster)  [unwired: 1 in, 1 out]
                }
                frame "Velocity" {
                  n174 = property on="Index" class="Ring (strict)"(error in=w606, "DisabledEnum"=T11."Disabled and Grayed Out" ("Disabled")) -> (error out=w608:errorcluster)  [unwired: 1 in, 1 out]
                }
                frame "Version" {
                  n175 = property on="Index" class="Ring (strict)"(error in=w610, "DisabledEnum"=T11."Disabled and Grayed Out" ("Disabled")) -> (error out=w609:errorcluster)  [unwired: 1 in, 1 out]
                }
              }
            }
            event "SetGet": Value Change {
              n176 = event-data() -> ()  [unwired: 1 in, 6 out]
              n177 = property on="Function" class="Enum (strict)"() -> ("Value"=w625:T1)  [unwired: 2 in, 2 out]
              n178 = case shown="\"Version\"" w625 {
                tunnel: w618 -> [w629 w633 w637 w641 w645 w649]
                tunnel: [FALSE TRUE TRUE FALSE FALSE FALSE] -> w623
                tunnel: [TRUE TRUE TRUE FALSE TRUE FALSE] -> w622
                tunnel: [FALSE FALSE FALSE TRUE FALSE FALSE] -> w621
                tunnel: [w629 w633 w637 w641 w645 w649] -> w619
                frame "Serial Number", Default {
                }
                frame "Temperature" {
                }
                frame "Unit Adress" {
                }
                frame "Calibration" {
                }
                frame "Velocity" {
                }
                frame "Version" {
                }
              }
              n179 = property on="Index" class="Ring (strict)"(error in=w619, "Visible"=w623) -> (error out=w624:errorcluster)  [unwired: 1 in, 1 out]
              n180 = property on="Value" class="DigNum (strict)"(error in=w624, "Visible"=w622) -> (error out=w620:errorcluster)  [unwired: 1 in, 1 out]
              n181 = property on="Value 1/2" class="Enum (strict)"(error in=w620, "Visible"=w621) -> (error out=w617:errorcluster)  [unwired: 1 in, 1 out]
            }
            event "Set Param.": Value Change {
              n182 = event-data() -> ()  [unwired: 1 in, 6 out]
              n183 = property on="Serial Status" class="Bool (strict)"(error in=w654) -> (error out=w653:errorcluster, "Value"=w658:bool)  [unwired: 1 in, 1 out]
              n184 = case shown="True" w658 {
                tunnel: w653 -> [w670 w680]
                tunnel: [w669 w675] -> w656
                frame False {
                  n185 = call "Display Message to User4"("error in (no error)"=w670) -> ("error out"=w669:errorcluster)  [unwired: 9 in, 1 out]
                }
                frame True {
                  n186 = property on="Speed control" class="Bool (strict)"(error in=w680, "Visible"=FALSE) -> (error out=w678:errorcluster)  [unwired: 1 in, 1 out]
                  n187 = case shown="47" "Param to Set" {
                    tunnel: [w736 w740 w744] -> w698
                    tunnel: w678 -> [w735 w739 w743]
                    tunnel: [w735 w739 w743] -> w686
                    frame 95, Default {
                      n188 = call <vilib>:"Application Directory.vi"() -> ("Application Directory"=w738:path)
                      n189 = Build Path(base path=w738, name or relative path="data\\Marvin_EBAY_params_RRPAR000017_95_v0.2.txt") -> (appended path=w736:path)
                    }
                    frame 63 {
                      n190 = call <vilib>:"Application Directory.vi"() -> ("Application Directory"=w742:path)
                      n191 = Build Path(base path=w742, name or relative path="data\\Marvin_AHU_params_RRPAR000016_63_v0.2.txt") -> (appended path=w740:path)
                    }
                    frame 47 {
                      n192 = call <vilib>:"Application Directory.vi"() -> ("Application Directory"=w746:path)
                      n193 = Build Path(base path=w746, name or relative path="data\\Marvin_AHU_params_RRPAR000015_47_v0.2.txt") -> (appended path=w744:path)
                    }
                  }
                  n194 = property on="read buffer" class="Str"(error in=w686, "Visible"=TRUE) -> (error out=w682:errorcluster)  [unwired: 1 in, 1 out]
                  n195 = property on="Array" class="Arr (strict)"(error in=w682, "Visible"=FALSE) -> (error out=w681:errorcluster)  [unwired: 1 in, 1 out]
                  n196 = property on="Horizontal Progress Bar" class="Slide (strict)"(error in=w681, "Visible"=TRUE, "Value"=u8 0 ("Horizontal Progress Bar")) -> (error out=w677:errorcluster)  [unwired: 1 in, 1 out]
                  n197 = call <vilib>:"Read Characters From File.vi"("file path (dialog if empty)"=w698) -> ("character string"=w699:string)  [unwired: 5 in, 3 out]
                  n198 = while {
                    shift-right: [w727] -> _
                    shift-left: w699 -> [w728]
                    shift-right: [w723] -> w684
                    shift-left: string[] [] -> [w724]
                    tunnel: w677 -> [w716]
                    tunnel: [w716] -> w696
                    stop <- w729 stop-if-true
                    n199 = Match Pattern(string=w728, regular expression="\r\n") -> (before substring=w725:string, after substring=w727:string, offset past match=w726:i32)  [unwired: 1 in, 1 out]
                    n200 = call <vilib>:"Trim Whitespace.vi"("string"=w725) -> ("trimmed string"=w722:string)  [unwired: 1 in]
                    n201 = Equal?(x=w726, y=-1) -> (x = y?=w729:bool)
                    n202 = To Upper Case(1:w722) -> (0:w720:string)
                    n203 = String Length(string=w720) -> (length=w719:i32)
                    n204 = Greater?(x=w719, y=3) -> (0:w717:bool)
                    n205 = case shown="True" w717 {
                      tunnel: w724 -> [w731 w734]
                      tunnel: [w731 w733] -> w723
                      tunnel: w720 -> [_ w732]
                      frame False {
                      }
                      frame True {
                        n206 = Build Array (concatenate)(w734, w732) -> (w733:string[])
                      }
                    }
                  }
                  n207 = property on="VISA resource name" class="VISAName"(error in=w696) -> (error out=w689:errorcluster, "Value"=w674:refnum<visa-resource-name>)  [unwired: 1 in, 1 out]
                  n208 = Build Array (concatenate)(w684, string[] ["MT", "VR", "SN"] ("array")) -> (w693:string[])
                  n209 = Array Size(array=w693) -> (size(s)=w685:i32)
                  n210 = Bundle By Name(cluster=T12 {"Minimum"=0.0, "Maximum"=0.0, "Increment"=0.0} ("Data Entry Limits"), "Minimum"=0.0, "Maximum"=w685) -> (w691:T12)
                  n211 = property on="Horizontal Progress Bar" class="Slide (strict)"(error in=w689, "Data Range"=w691) -> (error out=w673:errorcluster)  [unwired: 1 in, 1 out]
                  n212 = property on="read buffer" class="Str"(error in=w673) -> (error out=w672:errorcluster, "Text.Scroll Position"=w671:u32)  [unwired: 1 in, 1 out]
                  n213 = for {
                    tunnel: w693 -> [w707] mode=indexing
                    tunnel: w674 -> [w713]
                    tunnel: w672 -> [w712]
                    tunnel: [w704] -> w676
                    tunnel: w671 -> [w703]
                    i -> [w702]
                    n214 = Concatenate Strings(w707, "\r\n" ("string")) -> (w705:string)
                    n215 = VISA Write(VISA resource name=w713, write buffer=w705, error in (no error)=w712) -> (error out=w711:errorcluster)  [unwired: 2 out]
                    n216 = flat-sequence {
                      tunnel: w711 -> [w714]
                      tunnel: [w714] -> w704
                      frame #0 {
                        n217 = Wait (ms)(milliseconds to wait=u32 50) -> ()  [unwired: 1 out]
                      }
                    }
                    n218 = Add(x=w703, y=w702) -> (x+y=w701:u32)
                    n219 = feedback #2("") -> (w709:string)
                    n220 = Concatenate Strings(w709, w705) -> (w710:string)
                    n221 = feedback-in #2(w710) -> ()
                    n222 = property on="read buffer" class="Str"("Value"=w710, "Text.Scroll Position"=w701) -> ()  [unwired: 2 in, 2 out]
                    "Horizontal Progress Bar" <- w702
                  }
                  n223 = VISA Flush I/O Buffer(VISA resource name=w674, error in (no error)=w676) -> (error out=w675:errorcluster)  [unwired: 1 in, 1 out]
                }
              }
              n224 = property on="Serial Monitor" class="Bool (strict)"(error in=w656) -> (error out=w655:errorcluster, "Value"=w657:bool)  [unwired: 1 in, 1 out]
              n225 = case shown="False" w657 {
                tunnel: w655 -> [w667 w668]
                tunnel: [w665 w668] -> w651
                frame False {
                  n226 = property on="read buffer" class="Str"(error in=w667, "Visible"=FALSE) -> (error out=w666:errorcluster)  [unwired: 1 in, 1 out]
                  n227 = property on="Array" class="Arr (strict)"(error in=w666, "Visible"=TRUE) -> (error out=w665:errorcluster)  [unwired: 1 in, 1 out]
                }
                frame True {
                }
              }
              n228 = call "Display Message to User5"("error in (no error)"=w651) -> ("error out"=w650:errorcluster)  [unwired: 9 in, 1 out]
            }
            event "Help Button": Value Change {
              n229 = event-data() -> ()  [unwired: 1 in, 6 out]
              n230 = control-ref of="This VI"() -> (w754:refnum<vi>)
              n231 = property class="VI"(reference=w754, error in=w752, "FP:Transparency"=u8 25 ("Front Panel Window:Transparency")) -> (reference out=w748:refnum<vi>, error out=w751:errorcluster)
              n232 = vi-ref "Help.vi"() -> (w758:refnum<vi>)
              n233 = invoke class="VI" method="FP.Open"(reference=w758, error in=w751, "Activate"=TRUE ("Activate?"), "State"=T13."Standard") -> (error out=w757:errorcluster)  [unwired: 1 in, 4 out]
              n234 = call "Help.vi"("error in"=w757) -> ("error out"=w750:errorcluster)  [unwired: 7 in]
              n235 = property class="VI"(reference=w748, error in=w750, "FP:Transparency"=u8 0 ("Front Panel Window:Transparency")) -> (error out=w749:errorcluster)  [unwired: 1 out]
            }
            event "Can Send": Value Change {
              w783 = u8 0 items=["STATUS"=128, "EXTENDED"=2, "RTR"=1, "DATA MSG"=0] ("MSGTYPE")
              w788 = u8 1 items=["Standart flag", "Extern flag"] ("Format")
              w787 = u8 0 items=["Data flag", "Remote flag"] ("Type")
              # "Send"
              n236 = event-data() -> ()  [unwired: 1 in, 6 out]
              n237 = In Range and Coerce(upper limit=u16 18001, x="Motor Speed RPM", lower limit=u16 0) -> (coerced(x)=w770:u16, In Range?=w768:bool)
              n238 = Not(x=w768) -> (.not. x?=w769:bool)
              n239 = Select(t=w770, s=w768, f=u16 0) -> (s? t:f=w772:u16)
              n240 = property on="UUT" class="DigNum (strict)"() -> ("Value"=w766:u8)  [unwired: 2 in, 2 out]
              n241 = Split Number(x=w772) -> (hi(x)=w775:u8, lo(x)=w776:u8)
              n242 = call "Display Message to User"("Enable"=w769) -> ()  [unwired: 9 in, 2 out]
              n243 = case shown="47" w766 {
                tunnel: [u32 417357607 u32 417349415 u32 417345319] -> w767
                frame 95, Default {
                }
                frame 63 {
                }
                frame 47 {
                }
              }
              n244 = case shown="95" w766 {
                tunnel: [w807 w816 w829] -> w781
                tunnel: w776 -> [w806 w815 w828]
                tunnel: w775 -> [w805 w814 w827]
                tunnel: "Motor Speed RPM" -> [w802 w811 _]
                frame 47, Default {
                  w804 = u8 0 ("element")
                  n245 = case shown="1, Default" w802 {
                    tunnel: [u8 1 ("element") u8 0 ("element")] -> w801
                    frame 1, Default {
                    }
                    frame 0 {
                    }
                  }
                  n246 = Build Array(u8 1 ("element"), w806, w805, w801, w804, w804, w804, w804) -> (w807:u8[])
                }
                frame 63 {
                  w812 = u8 0 ("element")
                  n247 = case shown="1, Default" w811 {
                    tunnel: [u8 1 ("element") u8 0 ("element")] -> w810
                    frame 1, Default {
                    }
                    frame 0 {
                    }
                  }
                  n248 = Build Array(u8 1 ("element"), w815, w814, w810, w812, w812, w812, w812) -> (w816:u8[])
                }
                frame 95 {
                  w825 = u8 0 ("element")
                  n249 = Boolean To (0,1)(Boolean="Speed control") -> (0, 1=w823:i16)
                  n250 = Boolean To (0,1)(Boolean="Motor Over Temp") -> (0, 1=w824:i16)
                  n251 = To Unsigned Byte Integer(number=w823) -> (unsigned 8bit integer=w820:u8)
                  n252 = To Unsigned Byte Integer(number=w824) -> (unsigned 8bit integer=w819:u8)
                  n253 = Build Array(u8 1 ("element"), w828, w827, w820, w819, w825, w825, w825) -> (w829:u8[])
                }
              }
              n254 = Array Size(array=w781) -> (size(s)=w786:i32)
              n255 = call "Array Data to Single Num in Hex.vi"("aDATA"=w781) -> ("Numeric"=→"Data Send":u64)  [unwired: 10 in]
              n256 = To Unsigned Byte Integer(number=w786) -> (unsigned 8bit integer=w784:u8)
              n257 = call "CANAnalData.vi"("ID"=w767, "Data"=w781, "Config"=w779) -> ()  [unwired: 4 in, 5 out]
              n258 = Bundle By Name(cluster=T10 {"ID"=0, "MSGTYPE"=0, "LEN"=0, "aDATA"=[]} ("MsgTX 2"), "ID"=w767, "MSGTYPE"=w783, "LEN"=w784, "aDATA"=w781) -> (w782:T10)
              n259 = Unbundle By Name(w782) -> ("ID"=w796:u32, "LEN"=w797:u8, "aDATA"=w798:u8[])  [unwired: 1 out]
              n260 = property class="Clust (strict)"(reference=w779) -> ("Value"=w795:T8)  [unwired: 1 in, 2 out]
              n261 = Bundle By Name(cluster=T14 {"ID"=0, "TimeStamp"=0, "TimeFlag"=0, "SendType"=0, "RemoteFlag"=0, "ExternFlag"=0, "DataLen"=0, "Data"=[], "Reserved"=[]} ("Send"), "ID"=w796, "RemoteFlag"=w787, "ExternFlag"=w788, "DataLen"=w797, "Data"=w798) -> (w793:T14)
              n262 = Unbundle By Name(w795) -> ("DevType"=w789:T2, "DevIndex"=w790:u32, "CanIndex"=w791:T3)
              n263 = Build Array(w793) -> (w792:T14[])
              n264 = call "VCI_Transmit.vi"("Buffer"=w792, "CANIndex"=w791, "DevIndex"=w790, "DevType"=w789) -> ()  [unwired: 1 in, 7 out]
            }
            event "Graph Button": Value Change {
              w837 = FALSE ("Visible")
              n265 = event-data() -> ()  [unwired: 1 in, 6 out]
              n266 = Not(x="Graph Button") -> (.not. x?=w852:bool)
              n267 = property on="Array" class="Arr (strict)"(error in=w848, "Visible"=w852) -> (error out=w851:errorcluster)  [unwired: 1 in, 1 out]
              n268 = property on="Waveform Chart" class="WFChart (strict)"(error in=w851, "Visible"="Graph Button") -> (error out=w847:errorcluster)  [unwired: 1 in, 1 out]
              n269 = property on="Serial Monitor" class="Bool (strict)"(error in=w847) -> (error out=w849:errorcluster, "Value"=w850:bool)  [unwired: 1 in, 1 out]
              n270 = case shown="True" w850 {
                tunnel: w849 -> [w860 w863]
                tunnel: [w858 w861] -> w835
                frame False {
                  n271 = property on="read buffer" class="Str"(error in=w860, "Visible"=FALSE) -> (error out=w858:errorcluster)  [unwired: 1 in, 1 out]
                }
                frame True {
                  n272 = property on="read buffer" class="Str"(error in=w863, "Visible"=TRUE) -> (error out=w865:errorcluster)  [unwired: 1 in, 1 out]
                  n273 = property on="Array" class="Arr (strict)"(error in=w865, "Visible"=FALSE) -> (error out=w861:errorcluster)  [unwired: 1 in, 1 out]
                }
              }
              n274 = property on="Serial Monitor" class="Bool (strict)"(error in=w835, "Value"=FALSE ("Serial Monitor")) -> (error out=w833:errorcluster)  [unwired: 1 in, 1 out]
              n275 = property on="Index" class="Ring (strict)"(error in=w833, "Visible"=w837) -> (error out=w844:errorcluster)  [unwired: 1 in, 1 out]
              n276 = property on="Value 1/2" class="Enum (strict)"(error in=w844, "Visible"=w837) -> (error out=w843:errorcluster)  [unwired: 1 in, 1 out]
              n277 = property on="Value" class="DigNum (strict)"(error in=w843, "Visible"=w837) -> (error out=w842:errorcluster)  [unwired: 1 in, 1 out]
              n278 = property on="SetGet" class="Enum (strict)"(error in=w842, "Visible"=w837) -> (error out=w841:errorcluster)  [unwired: 1 in, 1 out]
              n279 = property on="Serial Send" class="Bool"(error in=w841, "Visible"=w837) -> (error out=w839:errorcluster)  [unwired: 1 in, 1 out]
              n280 = property on="Clear Monitor" class="Bool"(error in=w839, "Visible"=w837) -> (error out=w838:errorcluster)  [unwired: 1 in, 1 out]
              n281 = property on="Function" class="Enum (strict)"(error in=w838, "Visible"=w837) -> (error out=w840:errorcluster)  [unwired: 1 in, 1 out]
              n282 = property on="Index" class="Ring (strict)"(error in=w840, "Visible"=w837) -> (error out=w845:errorcluster)  [unwired: 1 in, 1 out]
              n283 = property on="read buffer" class="Str"(error in=w845, "Visible"=w837) -> (error out=w836:errorcluster)  [unwired: 1 in, 1 out]
            }
            event "Serial Com": Value Change {
              n284 = event-data() -> ()  [unwired: 1 in, 6 out]
              n285 = property on="Serial Com" class="Bool"(error in=w870, "Visible"=FALSE) -> (error out=w869:errorcluster)  [unwired: 1 in, 1 out]
              n286 = property on="VISA resource name" class="VISAName"(error in=w869, "Visible"=TRUE) -> (error out=w867:errorcluster)  [unwired: 1 in, 1 out]
            }
            event "VISA resource name": Value Change {
              n287 = event-data() -> ()  [unwired: 1 in, 1 out]
              n288 = control-ref of="This VI"() -> (w880:refnum<vi>)
              n289 = call "Serial InitMarvin.vi"("error in (no error)"=w885, "VI reference (current VI)"=w880, "VISA Refnum in"="VISA resource name") -> ("error out"=w894:errorcluster, "Boolean"=w882:bool)  [unwired: 7 in]
              n290 = property on="Serial Status" class="Bool (strict)"(error in=w894, "Value"=w882) -> (error out=w888:errorcluster)  [unwired: 1 in, 1 out]
              n291 = property on="VISA resource name" class="VISAName"(error in=w888, "Visible"=FALSE) -> (error out=w887:errorcluster)  [unwired: 1 in, 1 out]
              n292 = property on="Serial Com" class="Bool"(error in=w887, "Visible"=TRUE) -> (error out=w879:errorcluster)  [unwired: 1 in, 1 out]
              n293 = call "Serial.vi"("error in (no error)"=w879, "Clear Log"=TRUE, "VISA resource name"="VISA resource name") -> ("error out"=w877:errorcluster)  [unwired: 6 in, 2 out]
              n294 = call <vilib>:"Clear Errors.vi"("error in (no error)"=w877) -> ("error out"=w884:errorcluster)  [unwired: 5 in, 1 out]
              n295 = case shown="True" w882 {
                tunnel: w884 -> [w895 w898]
                tunnel: [w895 w897] -> w883
                tunnel: "VISA resource name" -> [_ w896]
                frame False {
                }
                frame True {
                  n296 = VISA Flush I/O Buffer(VISA resource name=w896, error in (no error)=w898) -> (error out=w897:errorcluster)  [unwired: 1 in, 1 out]
                }
              }
            }
            event "Stop": Value Change {
              n297 = event-data() -> ()  [unwired: 1 in, 6 out]
              n298 = Flush Queue(queue=w904, error in (no error)=w903) -> (queue out=w902:refnum<queue>, error out=w901:errorcluster)  [unwired: 1 out]
              n299 = Release Queue(queue=w902, error in (no error)=w901) -> (error out=w900:errorcluster)  [unwired: 1 in, 2 out]
            }
            event "Refresh Button": Value Change {
              n300 = event-data() -> ()  [unwired: 1 in, 6 out]
              n301 = Release Queue(queue=w910, error in (no error)=w911) -> (error out=w909:errorcluster)  [unwired: 1 in, 2 out]
            }
          }
          n302 = Unbundle By Name(w228) -> ("status"=w234:bool)
          n303 = Or(x=w234, y=w226) -> (x .or. y?=w233:bool)
        }
        n304 = while {
          shift-right: [w99] -> _
          shift-left: w85 -> [w101]
          shift-right: [w97] -> _
          shift-left: _ -> [w98]
          shift-right: [w94] -> _
          shift-left: dbl[] [] -> [w93]
          shift-right: [w91] -> _
          shift-left: w84 -> [w91]
          stop <- w100 stop-if-true
          n305 = Dequeue Element(queue=w101, error in (no error)=w91) -> (queue out=w99:refnum<queue>, element=w92:T9, error out=w100:errorcluster)  [unwired: 1 in, 1 out]
          n306 = for {
            tunnel: [w221] -> w96 mode=indexing
            tunnel: w92 -> [w220] mode=indexing
            tunnel: [w219] -> w95 mode=indexing
            n307 = Unbundle By Name(w220) -> ("aDATA"=w219:u8[])
            n308 = call "Array Data to Single Num in Hex.vi"("aDATA"=w219) -> ("Numeric"=w221:u64)  [unwired: 10 in]
          }
          n309 = Build Array (concatenate)(w96, w98) -> (w97:u64[][])
          "Array" <- w97
          n310 = for {
            tunnel: w95 -> [w106] mode=indexing
            tunnel: [w104] -> w94
            tunnel: w93 -> [w103]
            tunnel: w92 -> [w102]
            i -> [w105]
            n311 = case shown="0, Default" w105 {
              tunnel: w106 -> [w145 w182 w214]
              tunnel: [w119 w177 w209] -> w104
              tunnel: w103 -> [w120 w177 w209]
              tunnel: w102 -> [w118 _ _]
              frame 0, Default {
                # "Frame ID\n0x18E1273F"
                n312 = Index Array(array=w145, index #1=0 ("index"), index #2=1 ("index"), index #3=2 ("index"), index #4=3 ("index"), index #5=4 ("index"), index #6=5 ("index"), index #7=6 ("index"), index #8=7 ("index")) -> (element #1=w129:u8, element #2=w131:u8, element #3=w132:u8, element #4=w136:u8, element #5=w139:u8, element #6=w143:u8, element #7=w144:u8, element #8=w142:u8)
                n313 = Join Numbers(hi=w144, lo=w143) -> ((hi.lo)=w163:u16)
                n314 = Join Numbers(hi=w132, lo=w131) -> ((hi.lo)=w133:u16)
                n315 = Number To Hexadecimal String(2:w139) -> (0:w140:string)  [unwired: 1 in]
                n316 = Number To Hexadecimal String(2:w163) -> (0:w162:string)  [unwired: 1 in]
                n317 = Number To Hexadecimal String(2:w129) -> (0:w130:string)  [unwired: 1 in]
                n318 = Number To Hexadecimal String(2:w133) -> (0:w134:string)  [unwired: 1 in]
                n319 = Number To Hexadecimal String(2:w136) -> (0:w137:string)  [unwired: 1 in]
                n320 = Number To Hexadecimal String(2:w142) -> (0:w156:string)  [unwired: 1 in]
                n321 = Hexadecimal String To Number(string=w140) -> (number=w141:u32)  [unwired: 2 in, 1 out]
                n322 = Hexadecimal String To Number(string=w162) -> (number=w161:u32)  [unwired: 2 in, 1 out]
                n323 = Hexadecimal String To Number(string=w130) -> (number=w127:u32)  [unwired: 2 in, 1 out]
                n324 = Hexadecimal String To Number(string=w134) -> (number=w135:u32)  [unwired: 2 in, 1 out]
                n325 = Hexadecimal String To Number(string=w137) -> (number=w138:u32)  [unwired: 2 in, 1 out]
                n326 = Hexadecimal String To Number(string=w156) -> (number=w155:u32)  [unwired: 2 in, 1 out]
                n327 = To Double Precision Float(number=u32 10 ("y")) -> (double precision float=w159:dbl)
                n328 = To Double Precision Float(number=w161) -> (double precision float=w158:dbl)
                n329 = To Double Precision Float(number=w141) -> (double precision float=w122:dbl)
                n330 = To Double Precision Float(number=w135) -> (double precision float=w115:dbl)
                "Motor Speed RPM" <- w115
                n331 = To Double Precision Float(number=w138) -> (double precision float=w124:dbl)
                n332 = To Double Precision Float(number=w155) -> (double precision float=→"DC Current":dbl)
                n333 = Divide(x=w158, y=w159) -> (x/y=→"DC Voltage":dbl)
                n334 = To Unsigned Word Integer(number=w127) -> (unsigned 16bit integer=→"ECS State":u16)
                n335 = Subtract(x=w122, y=50.0 ("x")) -> (x-y=→"Power transistor Heat sink Temp.":dbl)
                n336 = Subtract(x=w124, y=50.0 ("x")) -> (x-y=→"Motor Stator Temp.":dbl)
                n337 = Index Array(array=w118, index=0) -> (element=w116:T10)
                n338 = Unbundle By Name(w116) -> ("ID"=w108:u32)
                n339 = Equal?(x=u32 417408815, y=w108) -> (x = y?=w109:bool)
                n340 = Equal?(x=u32 417408831, y=w108) -> (x = y?=w111:bool)
                n341 = Equal?(x=u32 417408863, y=w108) -> (x = y?=w110:bool)
                n342 = Compound Arithmetic op=OR(w111, w110, w109) -> (w107:bool)
                n343 = case shown="True" w107 {
                  tunnel: w120 -> [w164 w167]
                  tunnel: [w164 w166] -> w119
                  tunnel: w115 -> [_ w165]
                  frame False {
                  }
                  frame True {
                    n344 = disable-structure shown="Disabled" {
                      disable-tunnel: w165 -> [w171 _]
                      frame Disabled {
                        n345 = call <vilib>:"Application Directory.vi"() -> ("Application Directory"=w169:path)
                        n346 = Build Path(base path=w169, name or relative path="RPM Log.lvm") -> (appended path=w170:path)
                        n347 = call "Write To Measurement File2"("Signals"=w171, "Filename"=w170) -> ()  [unwired: 15 in, 3 out]
                      }
                      frame Enabled {
                      }
                    }
                    n348 = Build Array (concatenate)(w165, w167) -> (w166:dbl[])
                    "Waveform Chart" <- w166
                  }
                }
              }
              frame 1 {
                # "Framde ID\n0x18E3273F"
                n349 = Index Array(array=w182, index #1=0 ("index"), index #2=1 ("index")) -> (element #1=w180:u8, element #2=w174:u8)
                n350 = property on="UUT" class="DigNum (strict)"() -> ("Value"=w172:u8)  [unwired: 2 in, 2 out]
                n351 = Number To Boolean Array(number=w180) -> (Boolean array=w179:bool[])
                n352 = Number To Boolean Array(number=w174) -> (Boolean array=w176:bool[])
                n353 = Boolean To (0,1)(Boolean=w176) -> (0, 1=w173:i16[])
                n354 = Boolean To (0,1)(Boolean=w179) -> (0, 1=w178:i16[])
                n355 = case shown="95" w172 {
                  tunnel: w173 -> [_ w183]
                  frame 0, Default {
                  }
                  frame 95 {
                    n356 = for {
                      tunnel: w183 -> [w188] mode=indexing
                      i -> [w184]
                      stop <- w186 stop-if-true
                      n357 = Not Equal To 0?(x=w188) -> (x != 0?=w187:bool)
                      n358 = case shown="0, Default" w184 {
                        tunnel: w187 -> [w189 w190]
                        frame 0, Default {
                          "Ambient Sensor temp" <- w189
                        }
                        frame 1 {
                          "Ambient Over temp" <- w190
                        }
                      }
                      n359 = Equal?(x=w184, y=1.0) -> (x = y?=w186:bool)
                    }
                  }
                }
                n360 = for {
                  tunnel: w178 -> [w192] mode=indexing
                  i -> [w193]
                  n361 = Not Equal To 0?(x=w192) -> (x != 0?=w191:bool)
                  n362 = case shown="0, Default" w193 {
                    tunnel: w191 -> [w194 w195 w196 w197 w198 w199 w200 w201]
                    frame 0, Default {
                      "Drive Sensor temp Failure" <- w194
                    }
                    frame 1 {
                      "Drive Over temperature" <- w195
                    }
                    frame 2 {
                      "Motor Sensor temp Fauilre" <- w196
                    }
                    frame 3 {
                      "Motor Over temperature" <- w197
                    }
                    frame 4 {
                      "Derated drive temp" <- w198
                    }
                    frame 5 {
                      "Under voltage/Over voltage" <- w199
                    }
                    frame 6 {
                      "Commutation err" <- w200
                    }
                    frame 7 {
                      "Speed error" <- w201
                    }
                  }
                }
              }
              frame 2 {
                # "Frame ID\n0x18E2273F"
                n363 = Index Array(array=w214, index #1=0 ("index"), index #2=1 ("index")) -> (element #1=w211:u8, element #2=w207:u8)
                n364 = disable-structure shown="Enabled" {
                  disable-tunnel: [w217 w218] -> w212
                  disable-tunnel: w211 -> [w216 w218]
                  frame Disabled {
                    n365 = Number To Hexadecimal String(2:w216) -> (0:w215:string)  [unwired: 1 in]
                    n366 = Hexadecimal String To Number(string=w215) -> (number=w217:u32)  [unwired: 2 in, 1 out]
                  }
                  frame Enabled {
                  }
                }
                n367 = Number To Hexadecimal String(2:w207) -> (0:w205:string)  [unwired: 1 in]
                n368 = Hexadecimal String To Number(string=w205) -> (number=w206:u32)  [unwired: 2 in, 1 out]
                n369 = To Double Precision Float(number=w206) -> (double precision float=w204:dbl)
                n370 = To Double Precision Float(number=w212) -> (double precision float=→"Motor Phase Current RMS":dbl)
                n371 = Subtract(x=w204, y=50.0) -> (x-y=→"Ambient Temperature":dbl)
              }
            }
          }
        }
      }
      frame "Stop" {
        n372 = Release Queue(queue=w918, error in (no error)=w920) -> (error out=w919:errorcluster)  [unwired: 1 in, 2 out]
        n373 = flat-sequence {
          tunnel: w917 -> [w929]
          tunnel: [TRUE ("Stop")] -> w916
          frame #0 {
            w928 = u8[] [1, 0, 0, 0, 0, 0, 0, 0] ("Data 2")
            w931 = u8 0 items=["STATUS"=128, "EXTENDED"=2, "RTR"=1, "DATA MSG"=0] ("MSGTYPE")
            w936 = u8 1 items=["Standart flag", "Extern flag"] ("Format")
            w935 = u8 0 items=["Data flag", "Remote flag"] ("Type")
            n374 = property on="Serial Status" class="Bool (strict)"() -> ("Value"=w921:bool)  [unwired: 2 in, 2 out]
            n375 = property on="UUT" class="DigNum (strict)"() -> ("Value"=w923:u8)  [unwired: 2 in, 2 out]
            n376 = case shown="True" w921 {
              frame False {
              }
              frame True {
                n377 = property on="VISA resource name" class="VISAName"() -> ("Value"=w947:refnum<visa-resource-name>)  [unwired: 2 in, 2 out]
                n378 = VISA Close(VISA resource name=w947) -> ()  [unwired: 1 in, 1 out]
              }
            }
            n379 = case shown="95, Default" w923 {
              tunnel: [u32 417357607 u32 417349415 u32 417345319] -> w922
              frame 95, Default {
              }
              frame 63 {
              }
              frame 47 {
              }
            }
            n380 = property on="Graph Button" class="Bool (strict)"("Value"=FALSE ("Graph Button")) -> ()  [unwired: 2 in, 2 out]
            n381 = Array Size(array=w928) -> (size(s)=w934:i32)
            n382 = To Unsigned Byte Integer(number=w934) -> (unsigned 8bit integer=w932:u8)
            n383 = property on="Waveform Chart" class="WFChart (strict)"("Visible"=FALSE, "Value"=dbl[] [] ("Waveform Chart")) -> ()  [unwired: 2 in, 2 out]
            n384 = Bundle By Name(cluster=T10 {"ID"=0, "MSGTYPE"=0, "LEN"=0, "aDATA"=[]} ("MsgTX 2"), "ID"=w922, "MSGTYPE"=w931, "LEN"=w932, "aDATA"=w928) -> (w930:T10)
            n385 = call "CANAnalData.vi"("ID"=w922, "Data"=w928, "Config"=w929) -> ()  [unwired: 4 in, 5 out]
            n386 = call "Array Data to Single Num in Hex.vi"("aDATA"=w928) -> ("Numeric"=w927:u64)  [unwired: 10 in]
            n387 = property on="Data Send" class="DigNum (strict)"("Value"=w927) -> ()  [unwired: 2 in, 2 out]
            n388 = Unbundle By Name(w930) -> ("ID"=w944:u32, "LEN"=w945:u8, "aDATA"=w946:u8[])  [unwired: 1 out]
            n389 = property class="Clust (strict)"(reference=w929) -> ("Value"=w943:T8)  [unwired: 1 in, 2 out]
            n390 = Bundle By Name(cluster=T14 {"ID"=0, "TimeStamp"=0, "TimeFlag"=0, "SendType"=0, "RemoteFlag"=0, "ExternFlag"=0, "DataLen"=0, "Data"=[], "Reserved"=[]} ("Send"), "ID"=w944, "RemoteFlag"=w935, "ExternFlag"=w936, "DataLen"=w945, "Data"=w946) -> (w941:T14)
            n391 = Unbundle By Name(w943) -> ("DevType"=w937:T2, "DevIndex"=w938:u32, "CanIndex"=w939:T3)
            n392 = Build Array(w941) -> (w940:T14[])
            n393 = call "VCI_Transmit.vi"("Buffer"=w940, "CANIndex"=w939, "DevIndex"=w938, "DevType"=w937) -> ()  [unwired: 1 in, 7 out]
          }
          frame #1 {
          }
        }
      }
    }
  }
